vi "Read Dialog Listbox values.vi"(9 "Label.Text":string="Phase Shift, deg", 11 "module ref":refnum<vi>) -> (1 "Names, len":i32, 3 "Values":dbl[](array[numeric]))   [LabVIEW 2017]
panel:
  out "indices":i32[](array[numeric])
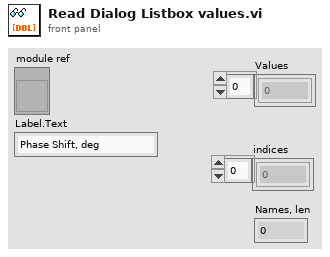
[diagram p1: front panel]
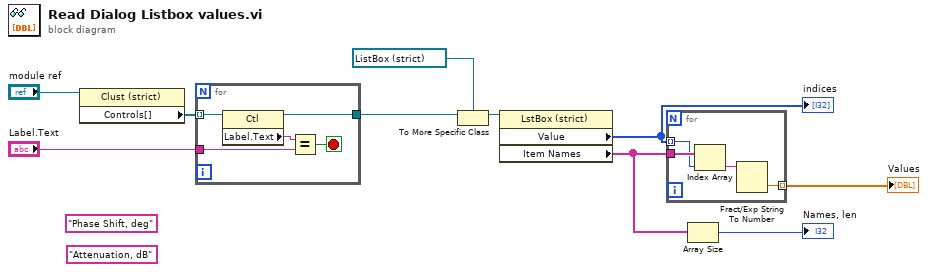
[diagram p0: block diagram]
diagram:
  (unwired) "Phase Shift, deg" ("Label.Text")
  (unwired) "Attenuation, dB" ("Label.Text")
  n1 = property class="Clust (strict)"(reference="module ref") -> ("Controls[]"=w10:refnum<vi>[])  [unwired: 1 in, 2 out]
  n2 = for {
    tunnel: w10 -> [w15] mode=indexing
    tunnel: "Label.Text" -> [w14]
    tunnel: [w11] -> w8
    stop <- w12 stop-if-true
    n3 = property class="Ctl"(reference=w15) -> (reference out=w11:refnum<vi>, "Label.Text"=w13:string)  [unwired: 1 in, 1 out]
    n4 = Equal?(x=w13, y=w14) -> (x = y?=w12:bool)
  }
  n5 = To More Specific Class(target class=refnum<vi> refnum ("Phase Shift, deg"), reference=w8) -> (specific class reference=w6:refnum<vi>)  [unwired: 1 in, 1 out]
  n6 = property class="LstBox (strict)"(reference=w6) -> ("Value"=w2:i32[], "Item Names"=w4:string[])  [unwired: 1 in, 2 out]
  "indices" <- w2
  n7 = for {
    tunnel: w2 -> [w18] mode=indexing
    tunnel: w4 -> [w19]
    tunnel: [w16] -> w1 mode=indexing
    n8 = Index Array(array=w19, index=w18) -> (element=w17:string)
    n9 = Fract/Exp String To Number(string=w17) -> (number=w16:dbl)  [unwired: 3 in, 1 out]
  }
  "Values" <- w1
  n10 = Array Size(array=w4) -> (size(s)=→"Names, len":i32)
